vi "PWM Write Duty.vi"(7 "GPIO #":T1=-1, 8 "error in (no error)":errorcluster, 10 "Duty % (0-1)":sgl, 11 "VisaComms in":refnum<class "VisaComms.lvclass">) -> (0 "error out":errorcluster, 3 "VisaComms out":refnum<class "VisaComms.lvclass">)   [LabVIEW 2024, in "CTI.lvlib" / "VisaComms.lvclass"]
uses:
  VisaComms.lvclass
  GPIO Number.ctl
  VisaComms.lvclass/VisaComms.ctl
  Clean Visa Errors.vi
  CTI.lvlib
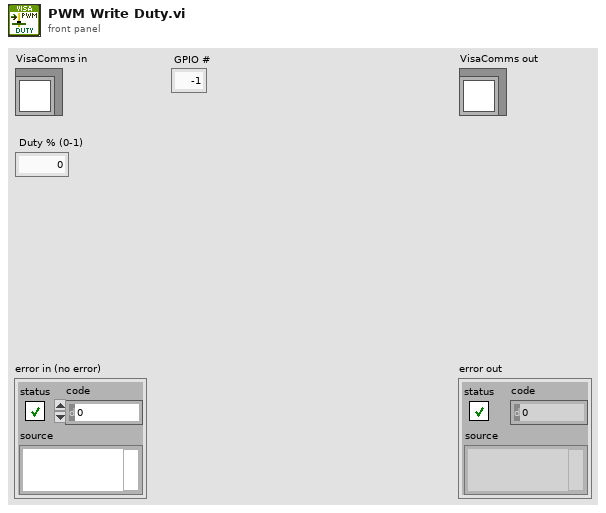
[diagram p1: front panel]
types:
  T1 = typedef "CTI.lvlib/GPIO Number.ctl" = i8
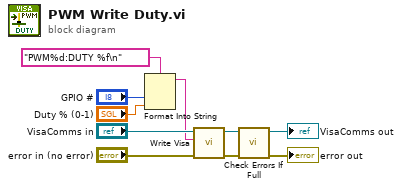
[diagram p0: block diagram]
diagram:
  n1 = Format Into String(format string="PWM%d:DUTY %f\n", "GPIO #", "Duty % (0-1)") -> (resulting string=w4:string)  [unwired: 2 in, 1 out]
  n2 = call "Write Visa.vi"("error in (no error)"="error in (no error)", "write buffer"=w4, "VisaComms in"="VisaComms in") -> ("error out"=w6:errorcluster, "VisaComms out"=w2:refnum<class "VisaComms.lvclass">)  [unwired: 6 in, 1 out]
  n3 = call "Check Errors If Full.vi"("error in (no error)"=w6, "VisaComms in"=w2) -> ("error out"=→"error out":errorcluster, "VisaComms out"=→"VisaComms out":refnum<class "VisaComms.lvclass">)  [unwired: 8 in]
